vi "EMD8216 point read.vi"(9 "point":u8, 10 "port":u8, 11 "CardID":u32) -> (1 "state":u8, 3 "error_code":u32)   [LabVIEW 2015, in "EMD8216_64.lvlib"]
doc: "EMD8216Status EMD8216_point_read(u32 CardID,u8 port,u8 point,u8 *state);"
uses:
  EMD8216_64.lvlib
  EMD8216_64.dll
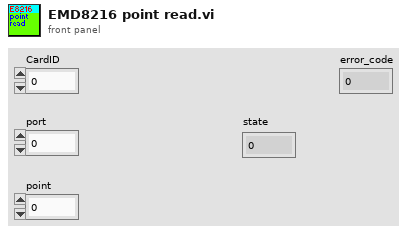
[diagram p1: front panel]
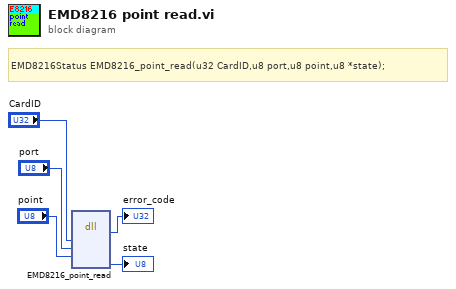
[diagram p0: block diagram]
diagram:
  # "EMD8216Status EMD8216_point_read(u32 CardID,u8 port,u8 point,u8 *state);"
  n1 = dll-call lib="C:/Users/jeff.lin.MINAIK/Documents/Soulkai/Labview/io/EMD8216_64/EMD8216_64/EMD8216_64.*" fn="EMD8216_point_read"("CardID"="CardID", "port"="port", "point"="point") -> ("return type"=→"error_code":u32, "state"=→"state":u8)  [unwired: 7 in, 2 out]
